vi "test class filtering.vi"() -> (0 "no err":errorcluster, 2 "OK":bool)   [LabVIEW 2025, in "NISE_CEF_Tests.lvlib"]
uses:
  NISE_CEF_Tests.lvlib
  Trunk/Configuration Framework/serializable node/NISE_CEF_serializable node.lvclass
  Trunk/ProjectTemplates/Source/Advanced Configurator/Classes/channel node/channel node.lvclass
  Trunk/ProjectTemplates/Source/Advanced Configurator/Classes/cRIO node/cRIO  node root.lvclass
  Trunk/ProjectTemplates/Source/Configuration Editor Framework/Classes/cRIO/cRIO.lvclass
  Trunk/ProjectTemplates/Source/Configuration Editor Framework/Classes/Channel/Channel.lvclass
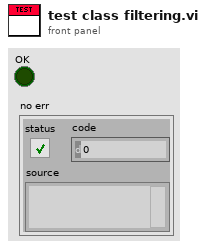
[diagram p1: front panel]
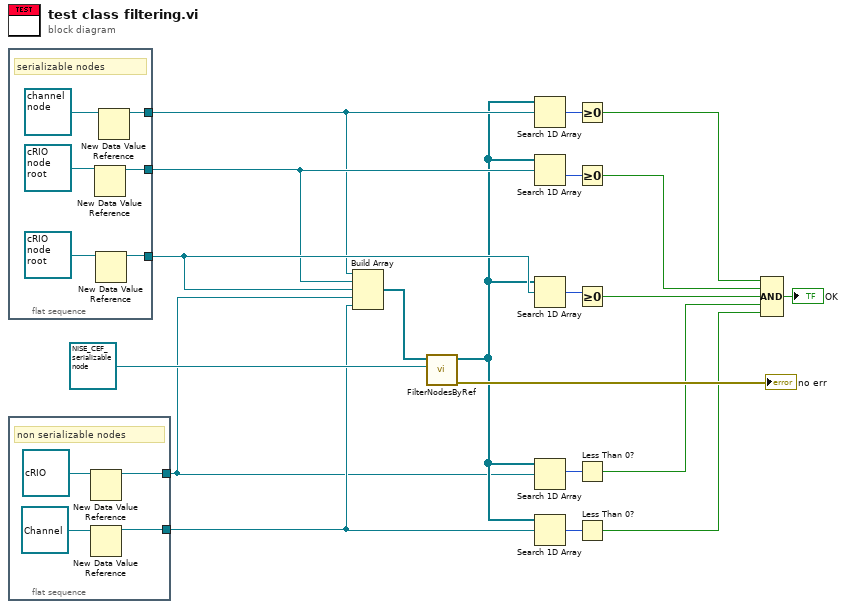
[diagram p0: block diagram]
diagram:
  n1 = flat-sequence {
    tunnel: [w23] -> w15
    tunnel: [w22] -> w16
    tunnel: [w21] -> w17
    frame #0 {
      # "serializable nodes"
      n2 = New Data Value Reference(data value=refnum<class "cRIO  node root.lvclass"> refnum ("cRIO  node root.lvclass")) -> (data value reference=w22:refnum<data-value>)  [unwired: 1 in, 1 out]
      n3 = New Data Value Reference(data value=refnum<class "cRIO  node root.lvclass"> refnum ("cRIO  node root.lvclass")) -> (data value reference=w21:refnum<data-value>)  [unwired: 1 in, 1 out]
      n4 = New Data Value Reference(data value=refnum<class "channel node.lvclass"> refnum ("channel node.lvclass")) -> (data value reference=w23:refnum<data-value>)  [unwired: 1 in, 1 out]
    }
  }
  n5 = flat-sequence {
    tunnel: [w28] -> w1
    tunnel: [w27] -> w2
    frame #0 {
      # "non serializable nodes"
      n6 = New Data Value Reference(data value=refnum<class "cRIO.lvclass"> refnum ("cRIO.lvclass")) -> (data value reference=w28:refnum<data-value>)  [unwired: 1 in, 1 out]
      n7 = New Data Value Reference(data value=refnum<class "Channel.lvclass"> refnum ("Channel.lvclass")) -> (data value reference=w27:refnum<data-value>)  [unwired: 1 in, 1 out]
    }
  }
  n8 = Build Array(w15, w16, w17, w1, w2) -> (w19:refnum<data-value>[])
  n9 = call "FilterNodesByRef.vi"("NISE_CEF_Node"=refnum<class "NISE_CEF_serializable node.lvclass"> refnum ("NISE_CEF_serializable node.lvclass"), "nodes"=w19) -> ("error out"=→"no err":errorcluster, "filtered nodes"=w3:refnum<data-value>[])  [unwired: 8 in]
  n10 = Search 1D Array(1D array=w3, element=w15) -> (index of element=w12:i32)  [unwired: 1 in]
  n11 = Search 1D Array(1D array=w3, element=w16) -> (index of element=w13:i32)  [unwired: 1 in]
  n12 = Search 1D Array(1D array=w3, element=w17) -> (index of element=w14:i32)  [unwired: 1 in]
  n13 = Search 1D Array(1D array=w3, element=w1) -> (index of element=w11:i32)  [unwired: 1 in]
  n14 = Search 1D Array(1D array=w3, element=w2) -> (index of element=w10:i32)  [unwired: 1 in]
  n15 = Greater Or Equal To 0?(x=w12) -> (x >= 0?=w5:bool)
  n16 = Greater Or Equal To 0?(x=w13) -> (x >= 0?=w6:bool)
  n17 = Greater Or Equal To 0?(x=w14) -> (x >= 0?=w7:bool)
  n18 = Less Than 0?(x=w11) -> (x < 0?=w8:bool)
  n19 = Less Than 0?(x=w10) -> (x < 0?=w9:bool)
  n20 = Compound Arithmetic op=AND(w5, w6, w7, w8, w9) -> (→"OK":bool)
